vi "StartImageAcquisition.vi"(10 "Camera mode (GrabToQueue)":T1=enum."GrabToQueue", 11 "Queue name (ImageAcqQueue)":string="ImageAcqQueue") -> (3 "Queue out":refnum<queue>)   [LabVIEW 2011]
uses:
  CmdData_NewFrame.ctl
  <vilib>/vision/Image Controls.llb/IMAQ Image.ctl
  CmdEnum_CameraFrameType.ctl
  CmdEnum_CameraIn.ctl
  CmdData_GrabParams.ctl
  qtrk/QTrk.llb/QTrkInstance.ctl
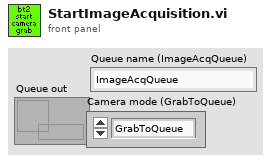
[diagram p1: front panel]
types:
  T1 = typedef "CmdEnum_CameraIn.ctl" = enum32{"Init", "Close", "ShowSettingsDialog", "EndGrab", "GrabZLUT", "GrabToTracker", "GrabToQueue", "AdjustROIs"}
  T2 = typedef "CmdData_GrabParams.ctl" = cluster{"QTrk Instance":T3, "Output Queue":refnum<queue>}
  T3 = typedef "QTrkInstance.ctl" = cluster{"QTrk Pointer":u64}
  T4 = typedef "CmdData_NewFrame.ctl" = cluster{"Buffer Image":T5, "Frame #":i32, "Hardware ROI Index":i32, "Timestamp":dbl, "Type":T6}
  T5 = typedef "IMAQ Image.ctl" = refnum<image>
  T6 = typedef "CmdEnum_CameraFrameType.ctl" = enum16{"Full", "HardwareROI", "EndGrabMarker"}
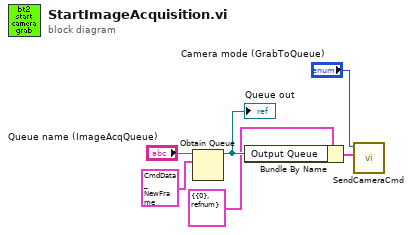
[diagram p0: block diagram]
diagram:
  n1 = Obtain Queue(name (unnamed)="Queue name (ImageAcqQueue)", element data type=T4 {"Buffer Image"=refnum, "Frame #"=0, "Hardware ROI Index"=0, "Timestamp"=0.0, "Type"=enum."Full"} ("Cluster")) -> (queue out=w3:refnum<queue>)  [unwired: 3 in, 2 out]
  "Queue out" <- w3
  n2 = Bundle By Name(cluster=T2 {"QTrk Instance"={"QTrk Pointer"=0}, "Output Queue"=refnum} ("GrabSessionParameters"), "Output Queue"=w3) -> (w1:T2)
  n3 = call "SendCameraCmd.vi"("Msg Data"=w1, "Camera cmd (SettingsDlg)"="Camera mode (GrabToQueue)") -> ()  [unwired: 10 in]
